vi "GrabWebCam_DALSA_IOS.vi"(0 "Session In":T3, 5 "Image In":T2, 7 "Trial Time":dbl, 9 "AVI Refnum":T1, 11 "error in":errorcluster) -> (4 "Session Out":T3, 6 "WebCam Img Out":T2, 8 "Buffer Number Out":u32, 15 "error out":errorcluster)   [LabVIEW 2020]
uses:
  <vilib>/userDefined/High Color/IMAQdx.ctl
  <vilib>/vision/Image Controls.llb/IMAQ Image.ctl
  <vilib>/vision/Avi.llb/IMAQ AVI2 Refnum.ctl
  <vilib>/vision/driver/NI_Vision_Acquisition_Software.lvlib
  <vilib>/vision/NI_Vision_Development_Module.lvlib
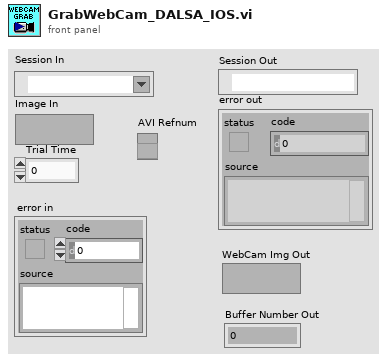
[diagram p1: front panel]
types:
  T1 = typedef "IMAQ AVI2 Refnum.ctl" = refnum<k20>
  T2 = typedef "IMAQ Image.ctl" = refnum<image>
  T3 = typedef "IMAQdx.ctl" = refnum<k21>
  T4 = cluster{"Desired Font (Application)":enum16{"User-specified Font", "Application Font", "System Font", "Dialog Font"}, "[User-specified Font]":cluster{"Font Name":string, "Size":i16, "Strikeout?":bool, "Italic?":bool, "Underline?":bool, "Outline?":bool, "Shadow?":bool, "Bold?":bool, "Rotation Angle":dbl}, "Horizontal Alignment":i16, "Vertical Alignment":i16}
  T5 = typedef "Image Type" = u32
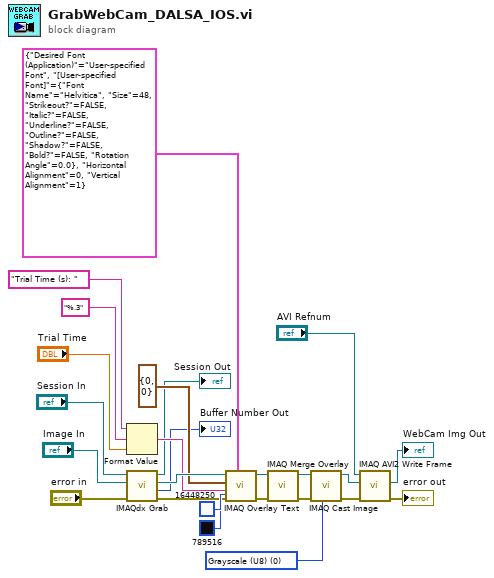
[diagram p0: block diagram]
diagram:
  w25 = T5 0 items=["Grayscale (U8)", "Grayscale (I16)", "Grayscale (SGL)", "Complex (CSG)", "RGB (U32)", "HSL (U32)", "RGB (U64)", "Grayscale (U16)"] ("Image Type")
  n1 = Format Value(string ("")="Trial Time (s): ", format string="%.3", value (0)="Trial Time") -> (output string=w12:string)
  n2 = call <vilib>:"IMAQdx Grab.vi"("error in"="error in", "Image In"="Image In", "Session In"="Session In") -> ("error out"=w13:errorcluster, "Buffer Number Out"=→"Buffer Number Out":u32, "Image Out"=w23:T2, "Session Out"=→"Session Out":T3)  [unwired: 5 in]
  n3 = call "IMAQ Overlay Text"("BG Color (Transparent)"=u32 789516, "Text Color (black)"=u32 16448250, "Font, Size & Style"=T4 {"Desired Font (Application)"=enum."User-specified Font", "[User-specified Font]"={"Font Name"="Helvitica", "Size"=48, "Strikeout?"=FALSE, "Italic?"=FALSE, "Underline?"=FALSE, "Outline?"=FALSE, "Shadow?"=FALSE, "Bold?"=FALSE, "Rotation Angle"=0.0}, "Horizontal Alignment"=0, "Vertical Alignment"=1}, "error in (no error)"=w13, "String"=w12, "Origin"=cluster{"X":i32, "Y":i32} {"X"=0, "Y"=0}, "Image"=w23) -> ("error out"=w17:errorcluster, "Image Out"=w18:T2)  [unwired: 3 in]
  n4 = call "IMAQ Merge Overlay"("error in (no error)"=w17, "Image Src"=w18) -> ("error out"=w15:errorcluster, "Image Dst Out"=w16:T2)  [unwired: 8 in]
  n5 = call "IMAQ Cast Image"("Image Type"=w25, "error in (no error)"=w15, "Image Src"=w16) -> ("error out"=w24:errorcluster, "Image Dst Out"=w14:T2)  [unwired: 7 in]
  n6 = call "IMAQ AVI2 Write Frame"("error in (no error)"=w24, "Image"=w14, "AVI Refnum"="AVI Refnum") -> ("error out"=→"error out":errorcluster, "Image Out (duplicate)"=→"WebCam Img Out":T2)  [unwired: 6 in, 1 out]
